vi "NiFPGA Read FIFO - I8.vi"(6 "Timeout":u32, 8 "error in (no error)":errorcluster, 9 "Number of Elements":u32, 10 "FIFO":u32, 11 "Session":u32) -> (0 "error out":errorcluster, 1 "Data":i8[](array[numeric]), 3 "Session Out":u32, 4 "Elements Remaining":u32)   [LabVIEW 2010, in "FPGA Interface Wrapper.lvlib"]
doc: "Reads from a FIFO of signed 8-bit integers."
uses:
  <userlib>/_FPGA Interface Advanced Tools/FPGA Interface Wrapper/FPGA Interface Wrapper.lvlib
  NiFpga.dll
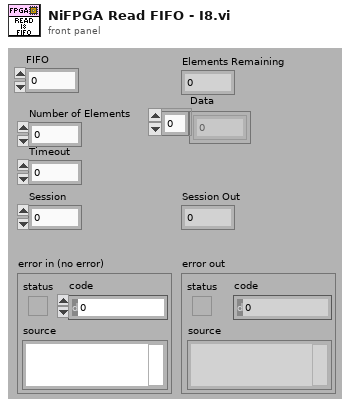
[diagram p1: front panel]
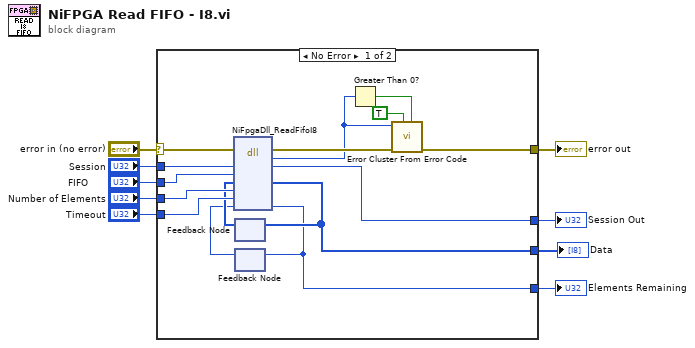
[diagram p0: block diagram]
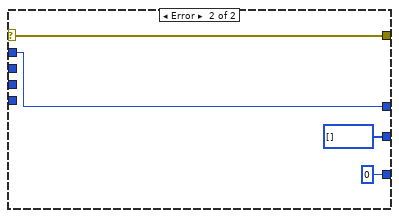
[diagram p2: hidden frame]
diagram:
  n1 = case shown="No Error" "error in (no error)" {
    selector: "error in (no error)" -> [w24 w27]
    tunnel: [w11 w27] -> w8
    tunnel: "Session" -> [w23 w28]
    tunnel: [w22 w28] -> w6
    tunnel: "FIFO" -> [w21 _]
    tunnel: "Number of Elements" -> [w20 _]
    tunnel: "Timeout" -> [w19 _]
    tunnel: [w15 u64 0 ("Elements Remaining")] -> w2
    tunnel: [w18 i8[] [] ("Data")] -> w1
    frame No Error {
      n2 = feedback #1() -> (w17:i8[])  [unwired: 1 in]
      n3 = feedback #2() -> (w16:u64)  [unwired: 1 in]
      n4 = dll-call lib="NiFpga.dll" fn="NiFpgaDll_ReadFifoI8"(error in=w24, "Session"=w23, "FIFO"=w21, "Data"=w17, "Number of Elements"=w20, "Timeout"=w19, "Elements Remaining"=w16) -> (error out=w12:errorcluster, "Status"=w10:i32, "Session"=w22:u32, "Data"=w18:i8[], "Elements Remaining"=w15:u64)  [unwired: 5 in, 1 out]
      n5 = feedback-in #1(w18) -> ()
      n6 = feedback-in #2(w15) -> ()
      n7 = Greater Than 0?(x=w10) -> (x > 0?=w13:bool)
      n8 = call <vilib>:"Error Cluster From Error Code.vi"("is warning? (False)"=w13, "show call chain? (False)"=TRUE, "error in (no error)"=w12, "error code (0)"=w10) -> ("error out"=w11:errorcluster)  [unwired: 5 in]
    }
    frame Error {
    }
  }
  "error out" <- w8
  "Session Out" <- w6
  "Elements Remaining" <- w2
  "Data" <- w1
